vi "Propagate Error.vi"(8 "error in (no error)":errorcluster, 11 "Propagate Error in":refnum<class "Propagate Error.lvclass">) -> (0 "error out":errorcluster, 3 "Propagate Error out":refnum<class "Propagate Error.lvclass">)   [LabVIEW 2021, in "LVCAM.lvlib" / "Propagate Error.lvclass"]
uses:
  Propagate Error.lvclass
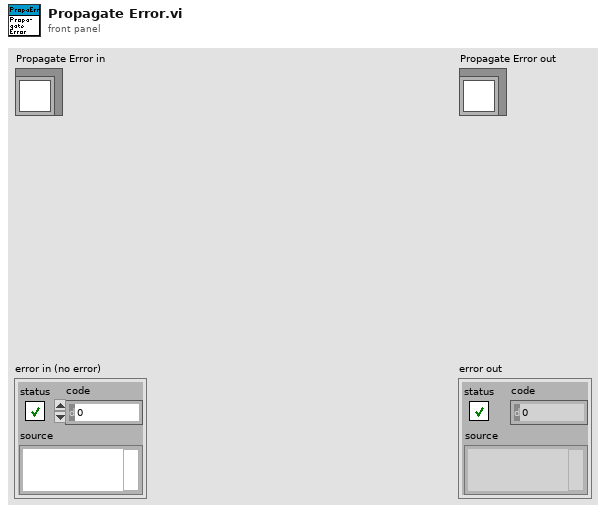
[diagram p1: front panel]
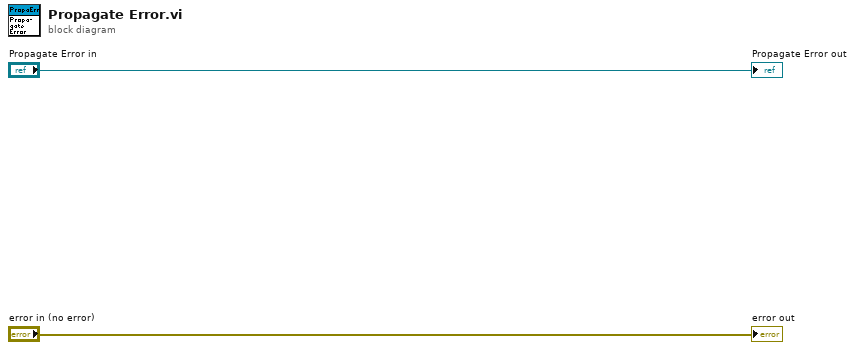
[diagram p0: block diagram]
diagram:
  "error out" <- "error in (no error)"
  "Propagate Error out" <- "Propagate Error in"
